vi "Gerador de sinais - Produtor consumidor.vi"() -> ()   [LabVIEW 2019]
doc: "[Covers: REQ08]\n[Covers: REQ04]\n[Covers: REQ05]\n[Covers: REQ06]\n[Covers: REQ03]"
uses:
  Estados - Consumidor.ctl
  Dados consumidor.ctl
  <vilib>/Utility/sysdir.llb/System Directory Type.ctl
  <vilib>/Waveform/WDTOps.llb/WDT Append Waveforms DBL.vi
  <vilib>/Waveform/WDTOps.llb/WDT Waveform Duration DBL.vi
  <vilib>/measure/NI_MABase.lvlib
panel:
  in  "Power":bool
  in  "Concatenar":bool
  in  "Adquirir entre cursores":bool
  in  "Deletar entre cursores":bool
  in  "Concatenar entre cursores":bool
  in  "Fase         º":dbl(slide) caption="Horizontal Slider" min=0.0 max=360.0 step=0.5 scale=0.0..360.0 scale format="%#.6g"
  in  "Offset":dbl(slide) caption="Vertical Slider" min=-10.0 max=10.0 step=0.01 scale=-10.0..10.0 scale format="%#2_2g"
  in  "Forma de onda":T1(ring) caption="Enum"
  in  "Tempo (Segundos)":dbl(knob)=1.0 min=0.0 max=1.0 scale=0.0..1.0
  in  "Abrir arquivo":bool
  in  "Salvar":bool
  out "Edição":waveform(dbl)(graph)
  out "Plot":waveform(dbl)(graph)
  in  "Razão cíclica (%)":dbl(knob)=50.0 min=0.0 max=100.0 step=0.5 scale=0.0..100.0
  in  "Amplitude":dbl(knob)=5.0 min=0.0 max=10.0 step=0.01 scale=0.0..10.0
  in  "Frequência":dbl(knob)=1.0 min=0.0 max=10.0 step=0.01 scale=0.0..10.0
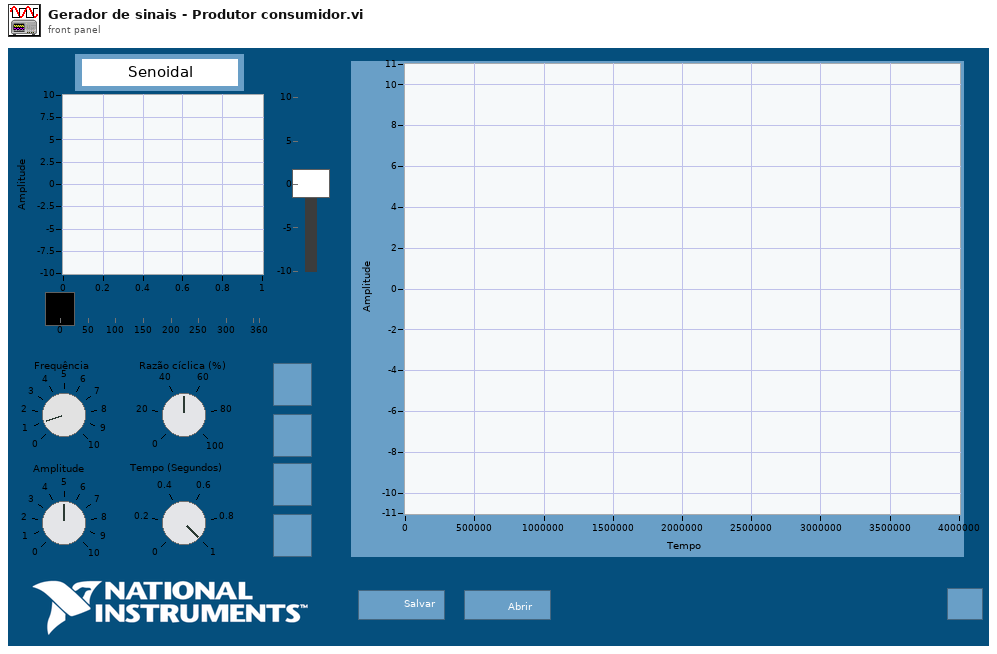
[diagram p1: front panel]
types:
  T1 = enum16{"Senoidal", "Triangular", "Quadrada", "Dente de Serra", "Trapezoidal"}
  T2 = typedef "Estados - Consumidor.ctl" = enum16{"Gerar onda", "Inicialização", "Parada", "Plotar", "Concatenar", "Concatenar - Cursores", "Adquirir entre Cursores", "Deletar entre Cursores", "Salvar onda", "Carregar onda", "Posicionar Cursores"}
  T3 = typedef "Dados consumidor.ctl" = cluster{"Onda gerada":cluster{"onda":waveform(dbl)}, "Onda modificada":cluster{"onda":waveform(dbl)}}
  T4 = typedef "Informações.ctl" = cluster{"Estados":T2, "Amplitude":dbl, "Informação\nde amostragem":cluster{"Fs":dbl, "#s":dbl}, "Frequência":dbl, "Offset":dbl, "Fase (Graus)":dbl, "Razão cíclica (%)":dbl, "Sinal":enum16{"Sine Wave", "Triangle Wave", "Square Wave", "Sawtooth Wave", "Trapezoidal Wave"}}
  T5 = enum8{"Enabled", "Disabled", "Disabled and Grayed Out"}
  T6 = enum16{"Sine Wave", "Triangle Wave", "Square Wave", "Sawtooth Wave", "Trapezoidal Wave"}
  T7 = enum16{"open", "open or create", "create or replace", "create", "open (read-only)"}
  T8 = typedef "System Directory Type.ctl" = i32
  T9 = cluster{"Amostras / s":dbl, "Quantidade\nde amostras":dbl}
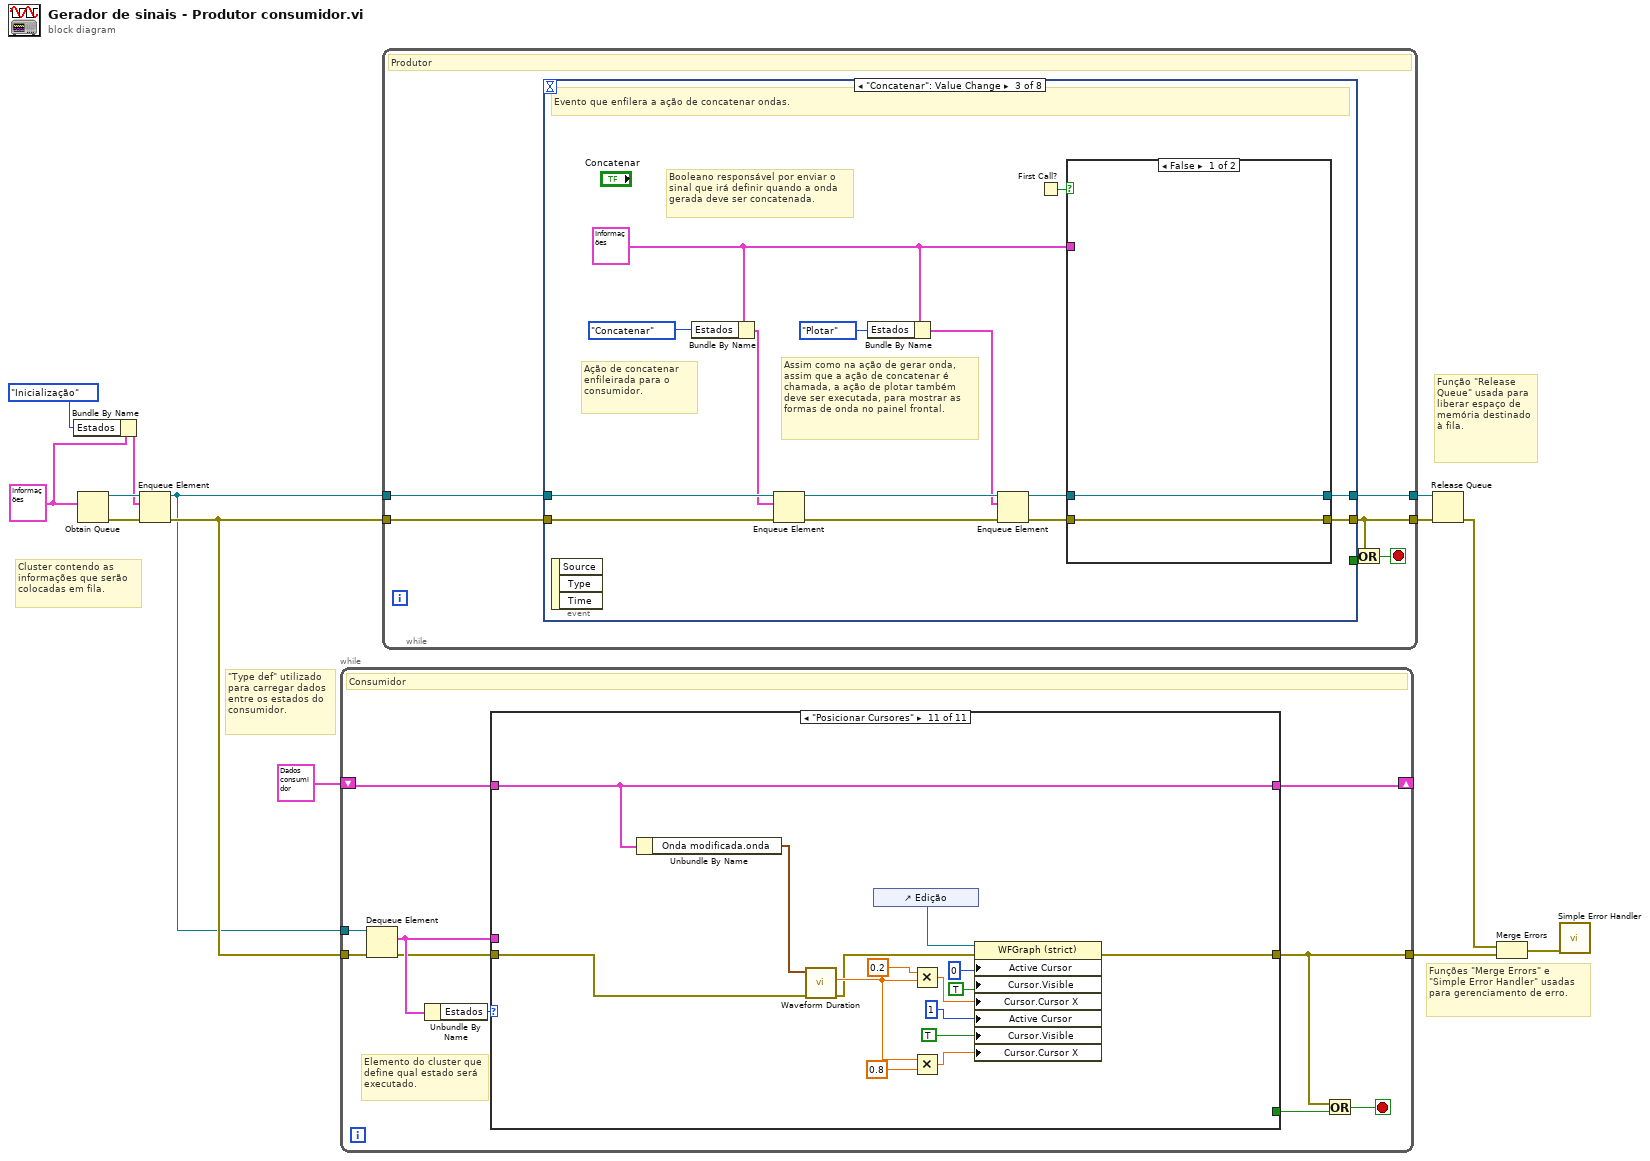
[diagram p0: block diagram]
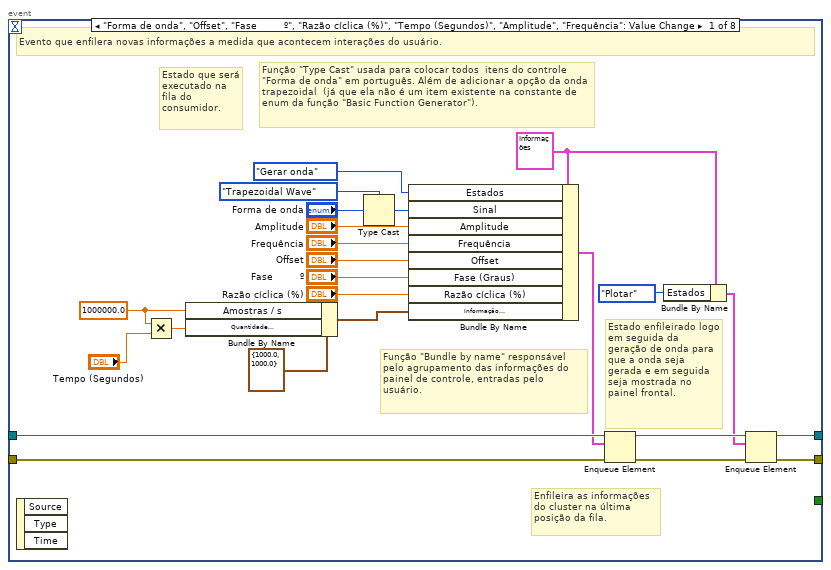
[diagram p2: hidden frame]
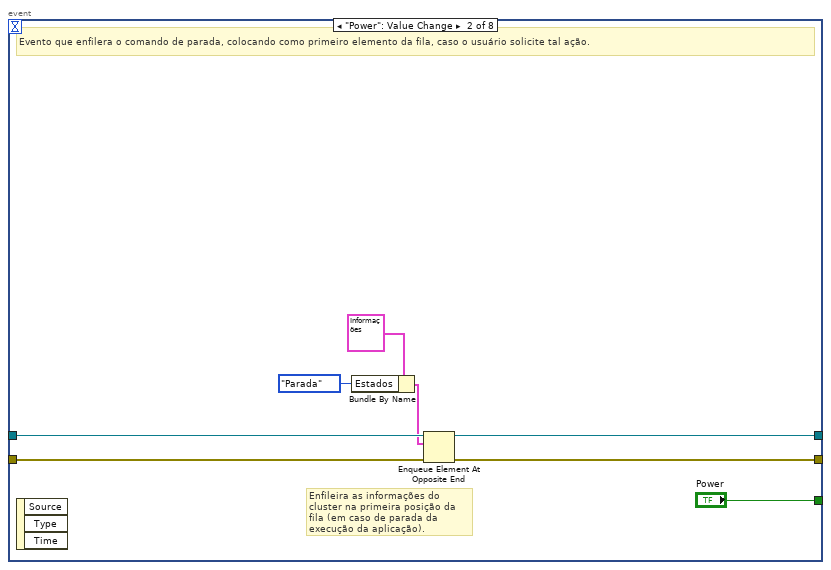
[diagram p3: hidden frame]
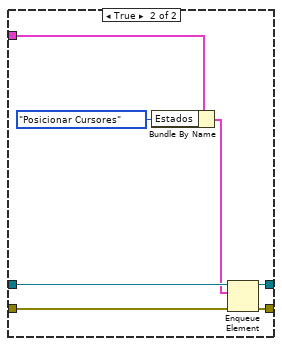
[diagram p4: hidden frame]
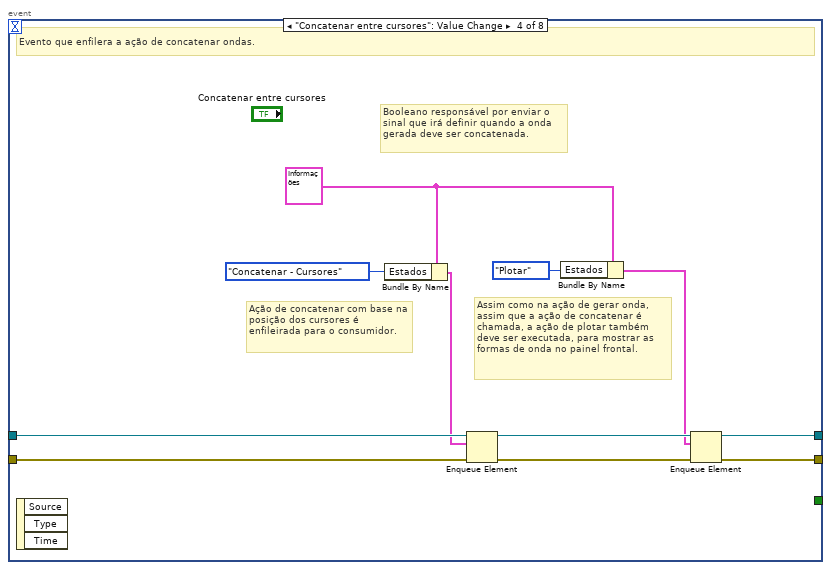
[diagram p5: hidden frame]
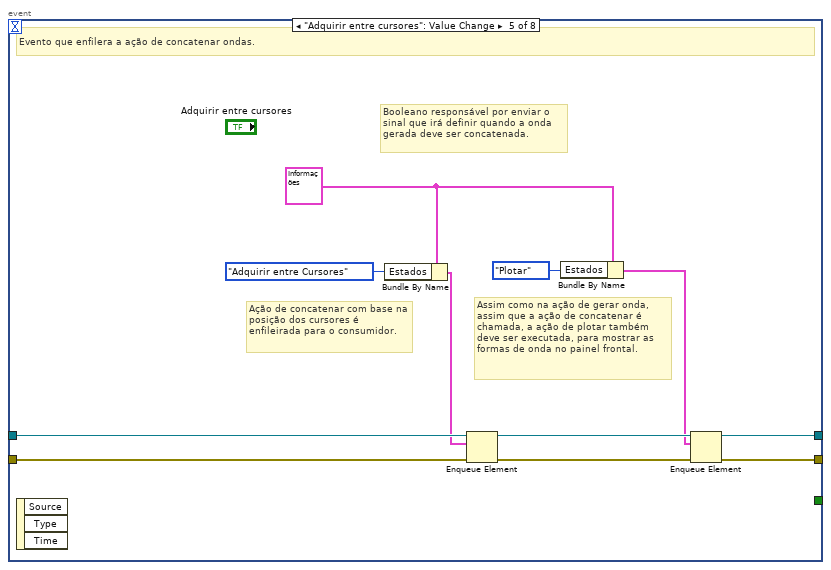
[diagram p6: hidden frame]
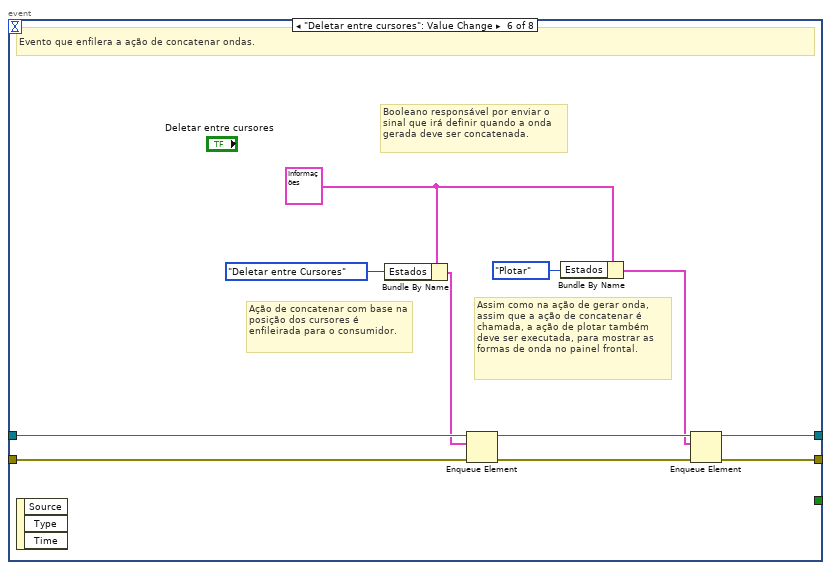
[diagram p7: hidden frame]
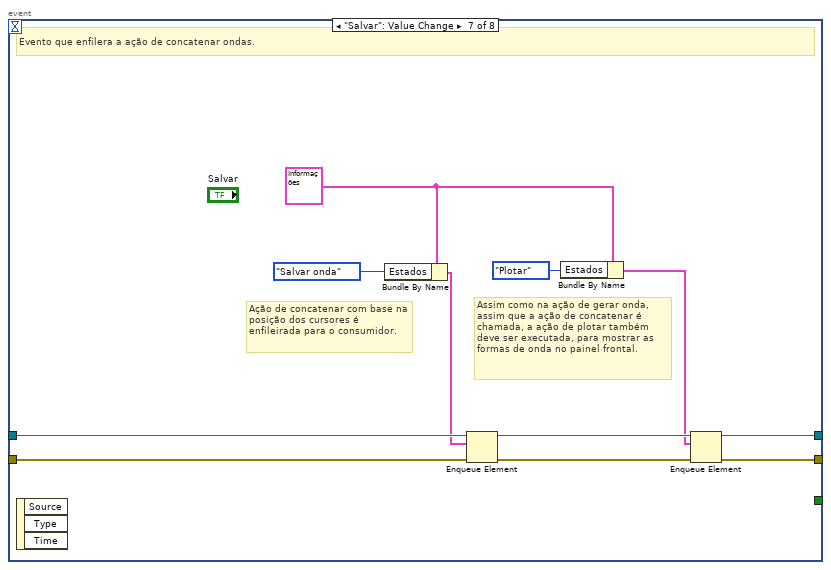
[diagram p8: hidden frame]
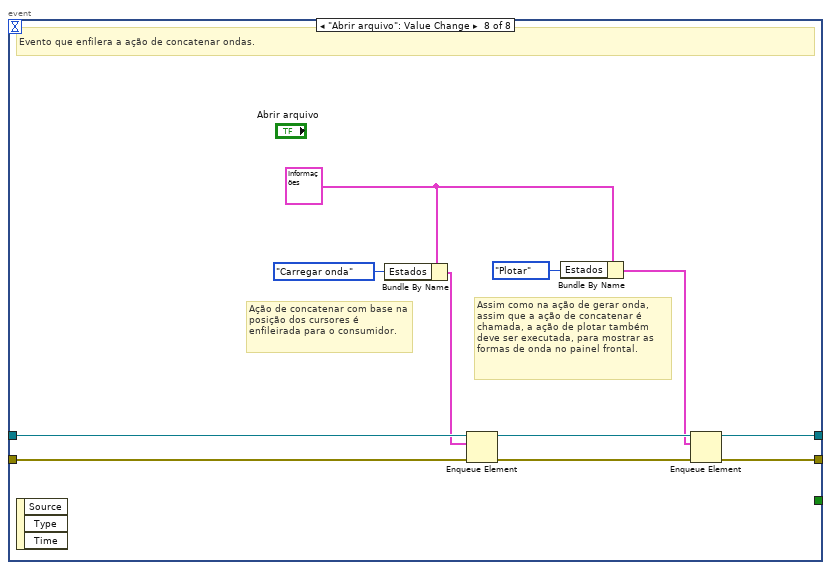
[diagram p9: hidden frame]
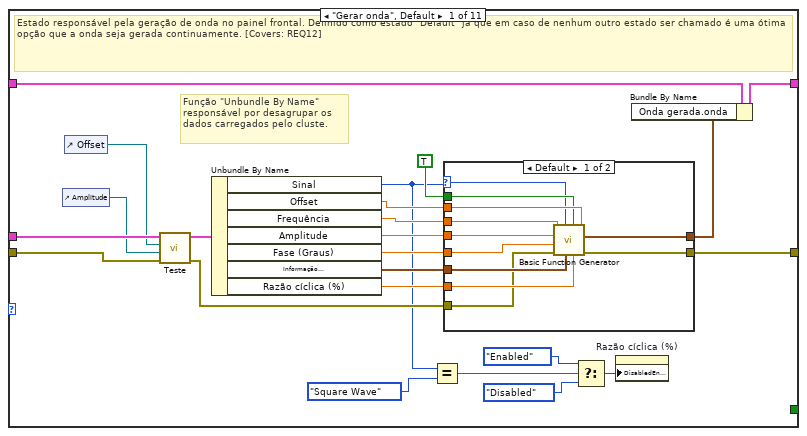
[diagram p10: hidden frame]
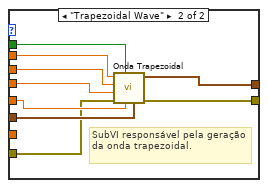
[diagram p11: hidden frame]
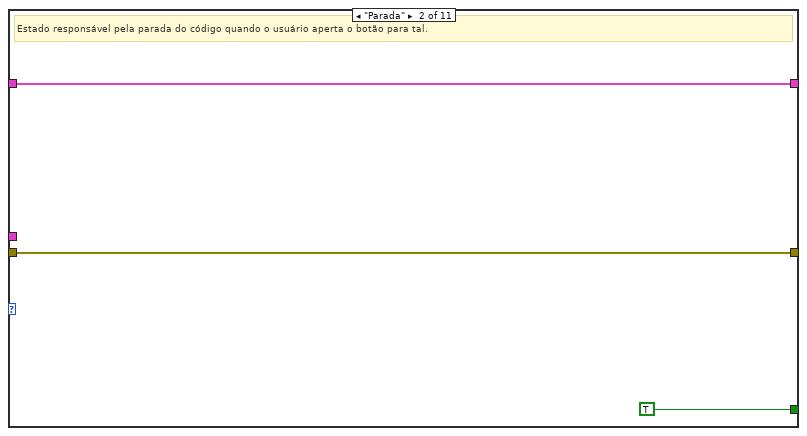
[diagram p12: hidden frame]
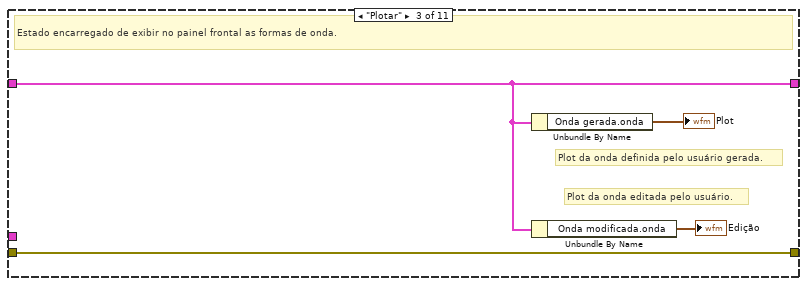
[diagram p13: hidden frame]
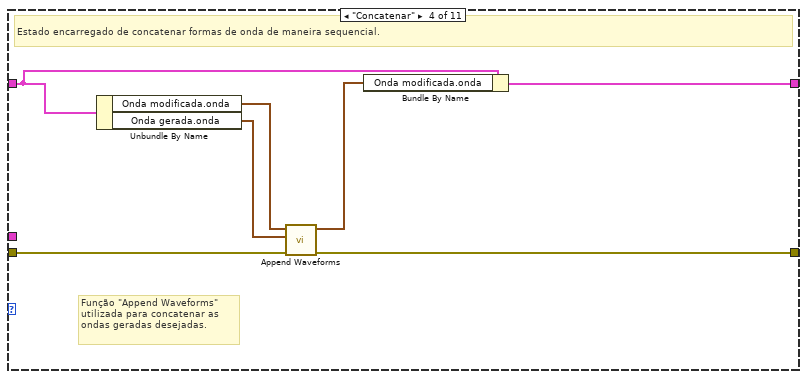
[diagram p14: hidden frame]
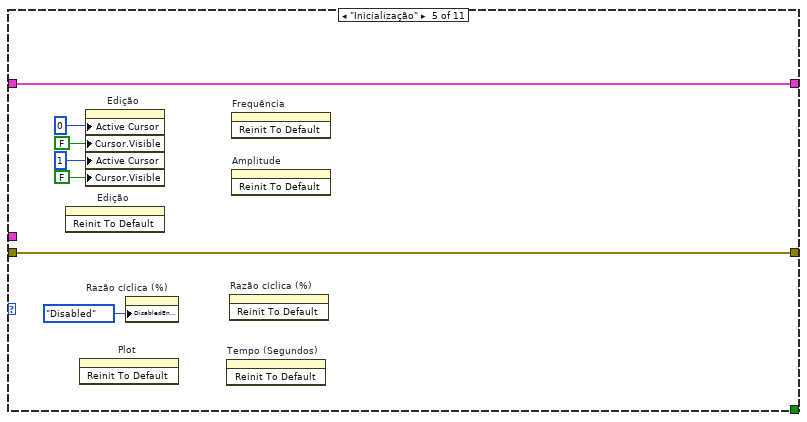
[diagram p15: hidden frame]
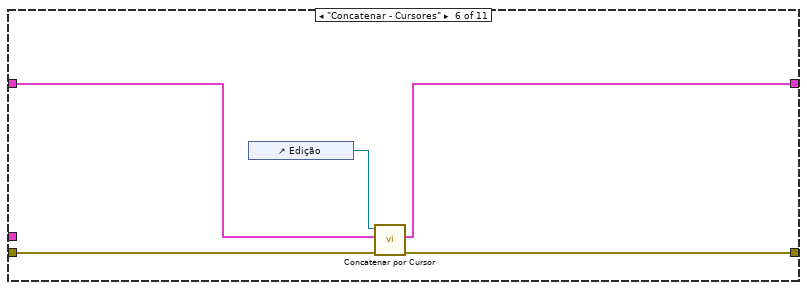
[diagram p16: hidden frame]
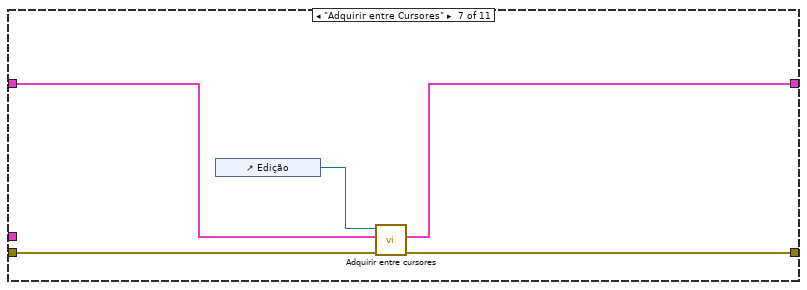
[diagram p17: hidden frame]
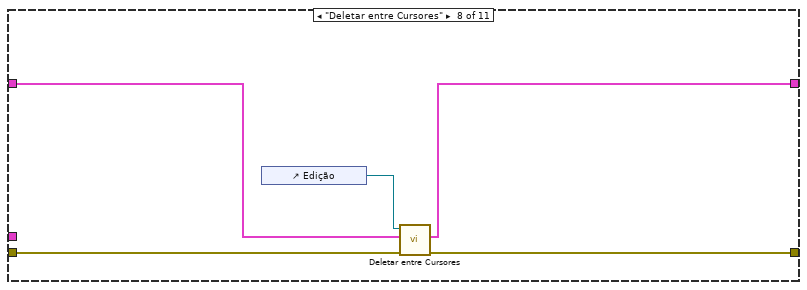
[diagram p18: hidden frame]
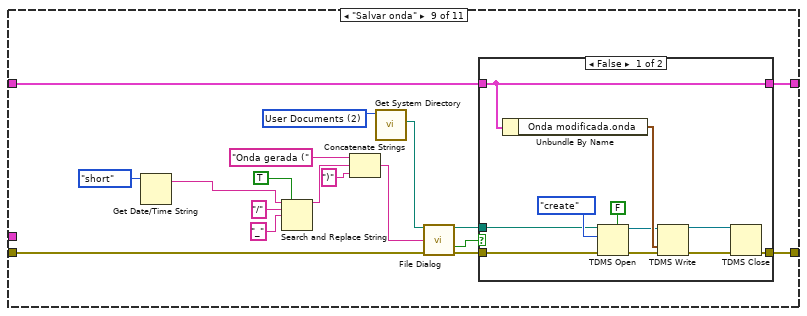
[diagram p19: hidden frame]
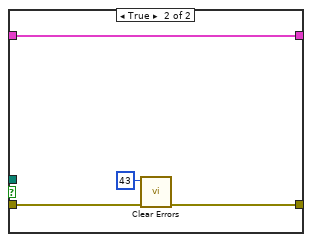
[diagram p20: hidden frame]
diagram:
  w2 = T4 {"Estados"=enum."Gerar onda", "Amplitude"=0.0, "Informação\nde amostragem"={"Fs"=1000.0, "#s"=1000.0}, "Frequência"=0.0, "Offset"=0.0, "Fase (Graus)"=0.0, "Razão cíclica (%)"=0.0, "Sinal"=enum."Sine Wave"}
  # "\"Type def\" utilizado para carregar dados entre os estados do consumidor."
  # "Funções \"Merge Errors\" e \"Simple Error Handler\" usadas para gerenciamento de erro."
  # "Função \"Release Queue\" usada para liberar espaço de memória destinado à fila."
  # "Cluster contendo as informações que serão colocadas em fila."
  n1 = Bundle By Name(cluster=w2, "Estados"=Estados_-_Consumidor."Inicialização") -> (w3:T4)
  n2 = Obtain Queue(element data type=w2) -> (queue out=w5:refnum<queue>, error out=w8:errorcluster)  [unwired: 4 in, 1 out]
  n3 = Enqueue Element(queue=w5, element=w3, error in (no error)=w8) -> (queue out=w4:refnum<queue>, error out=w6:errorcluster)  [unwired: 1 in, 1 out]
  n4 = while {
    tunnel: w4 -> [w16]
    tunnel: [w21] -> w10
    tunnel: w6 -> [w17]
    shift-right: [w15] -> _
    shift-left: T3 {"Onda gerada"={"onda"={"t0"=timestamp(0 s since 1904-01-01), "dt"=1.0, "Y"=[]}}, "Onda modificada"={"onda"={"t0"=timestamp(0 s since 1904-01-01), "dt"=1.0, "Y"=[]}}} ("Cluster 3") -> [w14]
    stop <- w19 stop-if-true
    # "Elemento do cluster que define qual estado será executado."
    # "Consumidor"
    n5 = Dequeue Element(queue=w16, error in (no error)=w17) -> (element=w22:T4, error out=w18:errorcluster)  [unwired: 1 in, 2 out]
    n6 = Unbundle By Name(w22) -> ("Estados"=w23:T2)
    n7 = case shown="\"Posicionar Cursores\"" w23 {
      tunnel: w22 -> [w46 _ _ _ _ _ _ _ _ _ _]
      tunnel: [_ TRUE _ _ _ _ _ _ _ _ _] -> w20
      tunnel: [w38 w67 w70 w74 w86 w90 w96 w98 w106 w137 w165] -> w21
      tunnel: w18 -> [w33 w67 w70 w77 w86 w91 w97 w99 w109 w140 w163]
      tunnel: [w36 w68 w71 w79 w87 w88 w94 w100 w103 w138 w167] -> w15
      tunnel: w14 -> [w37 w68 w71 w80 w87 w89 w95 w101 w107 w139 w167]
      frame "Gerar onda", Default {
        # "Função \"Unbundle By Name\" responsável por desagrupar os dados carregados pelo cluste."
        # "Estado responsável pela geração de onda no painel frontal. Definido como estado \"Default\" já que em caso de nenhum outro estado ser chamado é uma ótima opção que a onda seja gerada continuamente. [Covers: REQ12]"
        n8 = control-ref of="Amplitude"() -> (w31:refnum<vi>)
        n9 = control-ref of="Offset"() -> (w24:refnum<vi>)
        n10 = call "Teste.vi"("error in (no error)"=w33, "Amplitude Refnum"=w31, "Offset Refnum"=w24, 11:w46) -> ("error out"=w32:errorcluster, 3:w34:T4)  [unwired: 6 in]
        n11 = Unbundle By Name(w34) -> ("Sinal"=w25:T6, "Offset"=w45:dbl, "Frequência"=w44:dbl, "Amplitude"=w43:dbl, "Fase (Graus)"=w42:dbl, "Informação\nde amostragem"=w41:cluster{"Fs":dbl, "#s":dbl}, "Razão cíclica (%)"=w40:dbl)
        n12 = Equal?(x=w25, y=T6."Square Wave" ("Sinal")) -> (x = y?=w30:bool)
        n13 = case shown="Default" w25 {
          selector: w25 -> [w49 _]
          tunnel: w45 -> [w57 w60]
          tunnel: w44 -> [w56 w62]
          tunnel: w43 -> [w55 w61]
          tunnel: w42 -> [w54 w65]
          tunnel: w41 -> [w53 w64]
          tunnel: w40 -> [w52 _]
          tunnel: [w51 w63] -> w35
          tunnel: TRUE ("reset signal") -> [w50 w66]
          tunnel: [w48 w58] -> w38
          tunnel: w32 -> [w47 w59]
          frame Default {
            n14 = call <vilib>:"Basic Function Generator.vi"("offset"=w57, "square wave duty cycle (%)"=w52, "reset signal"=w50, "sampling info"=w53, "signal type"=w49, "error in (no error)"=w47, "phase"=w54, "amplitude"=w55, "frequency"=w56) -> ("error out"=w48:errorcluster, "signal out"=w51:waveform(dbl))  [unwired: 1 out]
          }
          frame "Trapezoidal Wave" {
            # "SubVI responsável pela geração da onda trapezoidal."
            n15 = call "Onda Trapezoidal.vi"("Informação\nde amostragem"=w64, "Fase (Graus)"=w65, "Reset do sinal"=w66, "Entrada de erro"=w59, "Amplitude"=w61, "Frequência"=w62, "Offset"=w60) -> ("Saída de erro"=w58:errorcluster, "Saída de sinal"=w63:waveform(dbl))  [unwired: 3 in]
          }
        }
        n16 = Select(t=T5."Enabled" ("Disabled"), s=w30, f=T5."Disabled" ("Disabled")) -> (s? t:f=w29:T5)
        n17 = property on="Razão cíclica (%)" class="Knob (strict)"("DisabledEnum"=w29) -> ()  [unwired: 2 in, 2 out]
        n18 = Bundle By Name(cluster=w37, "Onda gerada.onda"=w35) -> (w36:T3)
      }
      frame "Parada" {
        # "Estado responsável pela parada do código quando o usuário aperta o botão para tal."
      }
      frame "Plotar" {
        # "Plot da onda editada pelo usuário."
        # "Plot da onda definida pelo usuário gerada."
        # "Estado encarregado de exibir no painel frontal as formas de onda."
        n19 = Unbundle By Name(w71) -> ("Onda gerada.onda"=→"Plot":waveform(dbl))
        n20 = Unbundle By Name(w71) -> ("Onda modificada.onda"=→"Edição":waveform(dbl))
      }
      frame "Concatenar" {
        # "Função \"Append Waveforms\" utilizada para concatenar as ondas geradas desejadas."
        # "Estado encarregado de concatenar formas de onda de maneira sequencial."
        n21 = Unbundle By Name(w80) -> ("Onda modificada.onda"=w78:waveform(dbl), "Onda gerada.onda"=w76:waveform(dbl))
        n22 = call-poly <vilib>:"Append Waveforms.vi"("error in (no error)"=w77, "waveform B"=w76, "waveform A"=w78) -> ("error out"=w74:errorcluster, "waveform out"=w75:waveform(dbl))  [unwired: 7 in]
        n23 = Bundle By Name(cluster=w80, "Onda modificada.onda"=w75) -> (w79:T3)
      }
      frame "Inicialização" {
        n24 = invoke on="Edição" class="WFGraph (strict)" method="Reinit To Default"() -> ()  [unwired: 3 in, 3 out]
        n25 = invoke on="Plot" class="WFGraph (strict)" method="Reinit To Default"() -> ()  [unwired: 3 in, 3 out]
        n26 = property on="Edição" class="WFGraph (strict)"("Active Cursor"=u32 0, "Cursor.Visible"=FALSE, "Active Cursor"=u32 1, "Cursor.Visible"=FALSE) -> ()  [unwired: 2 in, 2 out]
        n27 = property on="Razão cíclica (%)" class="Knob (strict)"("DisabledEnum"=T5."Disabled" ("Disabled")) -> ()  [unwired: 2 in, 2 out]
        n28 = invoke on="Tempo (Segundos)" class="Knob (strict)" method="Reinit To Default"() -> ()  [unwired: 3 in, 3 out]
        n29 = invoke on="Razão cíclica (%)" class="Knob (strict)" method="Reinit To Default"() -> ()  [unwired: 3 in, 3 out]
        n30 = invoke on="Frequência" class="Knob (strict)" method="Reinit To Default"() -> ()  [unwired: 3 in, 3 out]
        n31 = invoke on="Amplitude" class="Knob (strict)" method="Reinit To Default"() -> ()  [unwired: 3 in, 3 out]
      }
      frame "Concatenar - Cursores" {
        n32 = control-ref of="Edição"() -> (w92:refnum<vi>)
        n33 = call "Concatenar por Cursor.vi"("error in"=w91, "Cluster 3"=w89, "WaveformGraph in"=w92) -> ("error out"=w90:errorcluster, "output cluster"=w88:T3)  [unwired: 7 in]
      }
      frame "Adquirir entre Cursores" {
        n34 = control-ref of="Edição"() -> (w93:refnum<vi>)
        n35 = call "Adquirir entre cursores.vi"("error in"=w97, "Input Cluster"=w95, "WaveformGraph in"=w93) -> ("error out"=w96:errorcluster, "Output Cluster"=w94:T3)  [unwired: 7 in]
      }
      frame "Deletar entre Cursores" {
        n36 = control-ref of="Edição"() -> (w102:refnum<vi>)
        n37 = call "Deletar entre Cursores.vi"("error in"=w99, "Cluster 3"=w101, "WaveformGraph in"=w102) -> ("error out"=w98:errorcluster, "output cluster"=w100:T3)  [unwired: 7 in]
      }
      frame "Salvar onda" {
        w110 = T8 2 items=["User Home"=0, "User Desktop"=1, "User Documents"=2, "User Application Data"=3, "User Preferences"=4, "User Temporary"=5, "Public Documents"=6, "Public Application Data"=7, "Public Preferences"=8, "Public Cache"=13, "System Core Libraries"=9, "System Installed Libraries"=10, "Application Files"=11, "Boot Volume Root"=12] ("system directory type")
        n38 = Get Date/Time String(date format (0)=enum16{"short", "long", "abbreviated"}."short") -> (date string=w115:string)  [unwired: 2 in, 1 out]
        n39 = Search and Replace String(replace all?=TRUE ("replace all? (F)"), input string=w115, search string="/", replace string="_" ("replace string (\"\")")) -> (result string=w120:string)  [unwired: 4 in, 3 out]
        n40 = Concatenate Strings("Onda gerada (" ("string"), w120, ")" ("string")) -> (w112:string)
        n41 = call <vilib>:"Get System Directory.vi"("system directory type"=w110) -> ("system directory"=w111:path)  [unwired: 10 in]
        n42 = call "File Dialog"("start path"=w111, "default name"=w112, "error in"=w109) -> ("selected path"=w108:path, "cancelled"=w105:bool, "error out"=w104:errorcluster)  [unwired: 9 in, 1 out]
        n43 = case shown="False" w105 {
          tunnel: w108 -> [w129 _]
          tunnel: w107 -> [w121 w135]
          tunnel: [w124 w132] -> w106
          tunnel: w104 -> [w122 w133]
          tunnel: [w121 w135] -> w103
          frame False {
            n44 = Unbundle By Name(w121) -> ("Onda modificada.onda"=w128:waveform(dbl))
            n45 = TDMS Open(5:FALSE ("create index file? (T)"), 8:w122, 10:T7."create" ("operation (0:open)"), 11:w129) -> (0:w127:errorcluster, 3:w126:refnum<k34>)  [unwired: 3 in]
            n46 = TDMS Write(0:w126, 9:w128, 11:w127) -> (4:w123:refnum<k34>, 15:w125:errorcluster)  [unwired: 3 in, 2 out]
            n47 = TDMS Close(8:w125, 11:w123) -> (0:w124:errorcluster)  [unwired: 1 out]
          }
          frame True {
            n48 = call <vilib>:"Clear Errors.vi"("error in (no error)"=w133, "specific error code to clear (0: all)"=43) -> ("error out"=w132:errorcluster)  [unwired: 4 in, 1 out]
          }
        }
      }
      frame "Carregar onda" {
        w143 = T8 2 items=["User Home"=0, "User Desktop"=1, "User Documents"=2, "User Application Data"=3, "User Preferences"=4, "User Temporary"=5, "Public Documents"=6, "Public Application Data"=7, "Public Preferences"=8, "Public Cache"=13, "System Core Libraries"=9, "System Installed Libraries"=10, "Application Files"=11, "Boot Volume Root"=12] ("system directory type")
        n49 = call <vilib>:"Get System Directory.vi"("system directory type"=w143) -> ("system directory"=w144:path)  [unwired: 10 in]
        n50 = call "File Dialog2"("start path"=w144, "error in"=w140) -> ("selected path"=w141:path, "cancelled"=w136:bool, "error out"=w142:errorcluster)  [unwired: 10 in, 1 out]
        n51 = case shown="False" w136 {
          tunnel: w142 -> [w145 w160]
          tunnel: w141 -> [w155 _]
          tunnel: w139 -> [w150 w158]
          tunnel: [w149 w158] -> w138
          tunnel: [w146 w159] -> w137
          frame False {
            n52 = TDMS Open(5:FALSE ("create index file? (T)"), 8:w145, 10:T7."open (read-only)" ("operation (0:open)"), 11:w155) -> (0:w154:errorcluster, 3:w153:refnum<k34>)  [unwired: 3 in]
            n53 = TDMS Read(0:w153, 11:w154, 12:waveform(dbl) {"t0"=timestamp(0 s since 1904-01-01), "dt"=1.0, "Y"=[]} ("Onda modificada.onda")) -> (4:w151:refnum<k34>, 10:w147:waveform(dbl), 15:w152:errorcluster)  [unwired: 5 in, 3 out]
            n54 = Bundle By Name(cluster=w150, "Onda modificada.onda"=w147) -> (w149:T3)
            n55 = TDMS Close(8:w152, 11:w151) -> (0:w146:errorcluster)  [unwired: 1 out]
          }
          frame True {
            n56 = call <vilib>:"Clear Errors.vi"("error in (no error)"=w160, "specific error code to clear (0: all)"=43) -> ("error out"=w159:errorcluster)  [unwired: 4 in, 1 out]
          }
        }
      }
      frame "Posicionar Cursores" {
        n57 = Unbundle By Name(w167) -> ("Onda modificada.onda"=w166:waveform(dbl))
        n58 = call-poly <vilib>:"Waveform Duration.vi"("error in (no error)"=w163, "waveform in"=w166) -> ("error out"=w164:errorcluster, "duration"=w174:dbl)  [unwired: 7 in, 1 out]
        n59 = control-ref of="Edição"() -> (w162:refnum<vi>)
        n60 = Multiply(x=0.2 ("y"), y=w174) -> (x*y=w176:dbl)
        n61 = Multiply(x=w174, y=0.8) -> (x*y=w175:dbl)
        n62 = property on="Property Node" class="WFGraph (strict)"(reference=w162, error in=w164, "Active Cursor"=u32 0, "Cursor.Visible"=TRUE, "Cursor.Cursor X"=w176, "Active Cursor"=u32 1, "Cursor.Visible"=TRUE, "Cursor.Cursor X"=w175) -> (error out=w165:errorcluster)  [unwired: 1 out]
      }
    }
    n63 = Or(x=w21, y=w20) -> (x .or. y?=w19:bool)
  }
  n64 = while {
    tunnel: w4 -> [w182]
    tunnel: [w178] -> w13
    tunnel: w6 -> [w181]
    tunnel: [w177] -> w12
    stop <- w179 stop-if-true
    # "Produtor"
    n65 = event shown="[2] \"Concatenar\": Value Change" {
      selector: _ -> [_ _ _ _ _ _ _ _]
      dyn-events: _ -> [_ _ _ _ _ _ _ _]
      timeout: _ -> [_ _ _ _ _ _ _ _]
      tunnel: w182 -> [w206 w212 w226 w245 w256 w267 w278 w289]
      tunnel: w181 -> [w205 w214 w228 w248 w259 w270 w281 w292]
      tunnel: [w197 w213 w216 w246 w257 w268 w279 w290] -> w177
      tunnel: [_ "Power" _ _ _ _ _ _] -> w180
      tunnel: [w195 w210 w215 w243 w254 w265 w276 w287] -> w178
      event "Forma de onda", "Offset", "Fase         º", "Razão cíclica (%)", "Tempo (Segundos)", "Amplitude", "Frequência": Value Change {
        w187 = 1000000.0 ("Quantidade\nde amostras")
        w194 = T4 {"Estados"=enum."Gerar onda", "Amplitude"=0.0, "Informação\nde amostragem"={"Fs"=1000.0, "#s"=1000.0}, "Frequência"=0.0, "Offset"=0.0, "Fase (Graus)"=0.0, "Razão cíclica (%)"=0.0, "Sinal"=enum."Sine Wave"}
        # "Estado enfileirado logo em seguida da geração de onda para que a onda seja gerada e em seguida seja mostrada no painel frontal."
        # "Função \"Type Cast\" usada para colocar todos  itens do controle \"Forma de onda\" em português. Além de adicionar a opção da onda trapezoidal  (já que ela não é um item existente na constante de enum da função \"Basic Function Generator\")."
        # "Estado que será executado na fila do consumidor."
        # "Enfileira as informações do cluster na última posição da fila."
        # "Função \"Bundle by name\" responsável pelo agrupamento das informações do painel de controle, entradas pelo usuário."
        # "Evento que enfilera novas informações a medida que acontecem interações do usuário."
        n66 = event-data() -> ()  [unwired: 1 in, 3 out]
        n67 = Multiply(x=w187, y="Tempo (Segundos)") -> (x*y=w188:dbl)
        n68 = Bundle By Name(cluster=T9 {"Amostras / s"=1000.0, "Quantidade\nde amostras"=1000.0} ("Informação\nde amostragem"), "Amostras / s"=w187, "Quantidade\nde amostras"=w188) -> (w189:T9)
        n69 = Type Cast(type=T6."Trapezoidal Wave" ("Forma de onda"), x="Forma de onda") -> (*(type *) &x=w198:T6)
        n70 = Bundle By Name(cluster=w194, "Estados"=Estados_-_Consumidor."Gerar onda", "Sinal"=w198, "Amplitude"="Amplitude", "Frequência"="Frequência", "Offset"="Offset", "Fase (Graus)"="Fase         º", "Razão cíclica (%)"="Razão cíclica (%)", "Informação\nde amostragem"=w189) -> (w200:T4)
        n71 = Enqueue Element(queue=w206, element=w200, error in (no error)=w205) -> (queue out=w196:refnum<queue>, error out=w204:errorcluster)  [unwired: 1 in, 1 out]
        n72 = Bundle By Name(cluster=w194, "Estados"=Estados_-_Consumidor."Plotar") -> (w193:T4)
        n73 = Enqueue Element(queue=w196, element=w193, error in (no error)=w204) -> (queue out=w195:refnum<queue>, error out=w197:errorcluster)  [unwired: 1 in, 1 out]
      }
      event "Power": Value Change {
        # "Enfileira as informações do cluster na primeira posição da fila (em caso de parada da execução da aplicação)."
        # "Evento que enfilera o comando de parada, colocando como primeiro elemento da fila, caso o usuário solicite tal ação."
        n74 = event-data() -> ()  [unwired: 1 in, 3 out]
        n75 = Bundle By Name(cluster=T4 {"Estados"=enum."Gerar onda", "Amplitude"=0.0, "Informação\nde amostragem"={"Fs"=1000.0, "#s"=1000.0}, "Frequência"=0.0, "Offset"=0.0, "Fase (Graus)"=0.0, "Razão cíclica (%)"=0.0, "Sinal"=enum."Sine Wave"}, "Estados"=Estados_-_Consumidor."Parada") -> (w211:T4)
        n76 = Enqueue Element At Opposite End(queue=w212, element=w211, error in (no error)=w214) -> (queue out=w210:refnum<queue>, error out=w213:errorcluster)  [unwired: 1 in, 1 out]
      }
      event "Concatenar": Value Change {
        w219 = T4 {"Estados"=enum."Gerar onda", "Amplitude"=0.0, "Informação\nde amostragem"={"Fs"=1000.0, "#s"=1000.0}, "Frequência"=0.0, "Offset"=0.0, "Fase (Graus)"=0.0, "Razão cíclica (%)"=0.0, "Sinal"=enum."Sine Wave"}
        # "Assim como na ação de gerar onda, assim que a ação de concatenar é chamada, a ação de plotar também deve ser executada, para mostrar as formas de onda no painel frontal."
        # "Ação de concatenar enfileirada para o consumidor."
        # "Booleano responsável por enviar o sinal que irá definir quando a onda gerada deve ser concatenada."
        # "Evento que enfilera a ação de concatenar ondas."
        n77 = event-data() -> ()  [unwired: 1 in, 3 out]
        n78 = Bundle By Name(cluster=w219, "Estados"=Estados_-_Consumidor."Concatenar") -> (w224:T4)
        n79 = Enqueue Element(queue=w226, element=w224, error in (no error)=w228) -> (queue out=w225:refnum<queue>, error out=w227:errorcluster)  [unwired: 1 in, 1 out]
        n80 = Bundle By Name(cluster=w219, "Estados"=Estados_-_Consumidor."Plotar") -> (w223:T4)
        n81 = Enqueue Element(queue=w225, element=w223, error in (no error)=w227) -> (queue out=w218:refnum<queue>, error out=w217:errorcluster)  [unwired: 1 in, 1 out]
        n82 = First Call?() -> (First Call?: T/F=w220:bool)
        n83 = case shown="False" w220 {
          tunnel: w219 -> [_ w236]
          tunnel: w218 -> [w230 w235]
          tunnel: w217 -> [w229 w234]
          tunnel: [w229 w233] -> w216
          tunnel: [w230 w232] -> w215
          frame False {
          }
          frame True {
            n84 = Bundle By Name(cluster=w236, "Estados"=Estados_-_Consumidor."Posicionar Cursores") -> (w231:T4)
            n85 = Enqueue Element(queue=w235, element=w231, error in (no error)=w234) -> (queue out=w232:refnum<queue>, error out=w233:errorcluster)  [unwired: 1 in, 1 out]
          }
        }
      }
      event "Concatenar entre cursores": Value Change {
        w240 = T4 {"Estados"=enum."Gerar onda", "Amplitude"=0.0, "Informação\nde amostragem"={"Fs"=1000.0, "#s"=1000.0}, "Frequência"=0.0, "Offset"=0.0, "Fase (Graus)"=0.0, "Razão cíclica (%)"=0.0, "Sinal"=enum."Sine Wave"}
        # "Assim como na ação de gerar onda, assim que a ação de concatenar é chamada, a ação de plotar também deve ser executada, para mostrar as formas de onda no painel frontal."
        # "Ação de concatenar com base na posição dos cursores é enfileirada para o consumidor."
        # "Booleano responsável por enviar o sinal que irá definir quando a onda gerada deve ser concatenada."
        # "Evento que enfilera a ação de concatenar ondas."
        n86 = event-data() -> ()  [unwired: 1 in, 3 out]
        n87 = Bundle By Name(cluster=w240, "Estados"=Estados_-_Consumidor."Concatenar - Cursores") -> (w242:T4)
        n88 = Enqueue Element(queue=w245, element=w242, error in (no error)=w248) -> (queue out=w244:refnum<queue>, error out=w247:errorcluster)  [unwired: 1 in, 1 out]
        n89 = Bundle By Name(cluster=w240, "Estados"=Estados_-_Consumidor."Plotar") -> (w241:T4)
        n90 = Enqueue Element(queue=w244, element=w241, error in (no error)=w247) -> (queue out=w243:refnum<queue>, error out=w246:errorcluster)  [unwired: 1 in, 1 out]
      }
      event "Adquirir entre cursores": Value Change {
        w251 = T4 {"Estados"=enum."Gerar onda", "Amplitude"=0.0, "Informação\nde amostragem"={"Fs"=1000.0, "#s"=1000.0}, "Frequência"=0.0, "Offset"=0.0, "Fase (Graus)"=0.0, "Razão cíclica (%)"=0.0, "Sinal"=enum."Sine Wave"}
        # "Assim como na ação de gerar onda, assim que a ação de concatenar é chamada, a ação de plotar também deve ser executada, para mostrar as formas de onda no painel frontal."
        # "Ação de concatenar com base na posição dos cursores é enfileirada para o consumidor."
        # "Booleano responsável por enviar o sinal que irá definir quando a onda gerada deve ser concatenada."
        # "Evento que enfilera a ação de concatenar ondas."
        n91 = event-data() -> ()  [unwired: 1 in, 3 out]
        n92 = Bundle By Name(cluster=w251, "Estados"=Estados_-_Consumidor."Adquirir entre Cursores") -> (w253:T4)
        n93 = Enqueue Element(queue=w256, element=w253, error in (no error)=w259) -> (queue out=w255:refnum<queue>, error out=w258:errorcluster)  [unwired: 1 in, 1 out]
        n94 = Bundle By Name(cluster=w251, "Estados"=Estados_-_Consumidor."Plotar") -> (w252:T4)
        n95 = Enqueue Element(queue=w255, element=w252, error in (no error)=w258) -> (queue out=w254:refnum<queue>, error out=w257:errorcluster)  [unwired: 1 in, 1 out]
      }
      event "Deletar entre cursores": Value Change {
        w262 = T4 {"Estados"=enum."Gerar onda", "Amplitude"=0.0, "Informação\nde amostragem"={"Fs"=1000.0, "#s"=1000.0}, "Frequência"=0.0, "Offset"=0.0, "Fase (Graus)"=0.0, "Razão cíclica (%)"=0.0, "Sinal"=enum."Sine Wave"}
        # "Assim como na ação de gerar onda, assim que a ação de concatenar é chamada, a ação de plotar também deve ser executada, para mostrar as formas de onda no painel frontal."
        # "Ação de concatenar com base na posição dos cursores é enfileirada para o consumidor."
        # "Booleano responsável por enviar o sinal que irá definir quando a onda gerada deve ser concatenada."
        # "Evento que enfilera a ação de concatenar ondas."
        n96 = event-data() -> ()  [unwired: 1 in, 3 out]
        n97 = Bundle By Name(cluster=w262, "Estados"=Estados_-_Consumidor."Deletar entre Cursores") -> (w264:T4)
        n98 = Enqueue Element(queue=w267, element=w264, error in (no error)=w270) -> (queue out=w266:refnum<queue>, error out=w269:errorcluster)  [unwired: 1 in, 1 out]
        n99 = Bundle By Name(cluster=w262, "Estados"=Estados_-_Consumidor."Plotar") -> (w263:T4)
        n100 = Enqueue Element(queue=w266, element=w263, error in (no error)=w269) -> (queue out=w265:refnum<queue>, error out=w268:errorcluster)  [unwired: 1 in, 1 out]
      }
      event "Salvar": Value Change {
        w273 = T4 {"Estados"=enum."Gerar onda", "Amplitude"=0.0, "Informação\nde amostragem"={"Fs"=1000.0, "#s"=1000.0}, "Frequência"=0.0, "Offset"=0.0, "Fase (Graus)"=0.0, "Razão cíclica (%)"=0.0, "Sinal"=enum."Sine Wave"}
        # "Assim como na ação de gerar onda, assim que a ação de concatenar é chamada, a ação de plotar também deve ser executada, para mostrar as formas de onda no painel frontal."
        # "Ação de concatenar com base na posição dos cursores é enfileirada para o consumidor."
        # "Evento que enfilera a ação de concatenar ondas."
        n101 = event-data() -> ()  [unwired: 1 in, 3 out]
        n102 = Bundle By Name(cluster=w273, "Estados"=Estados_-_Consumidor."Salvar onda") -> (w275:T4)
        n103 = Enqueue Element(queue=w278, element=w275, error in (no error)=w281) -> (queue out=w277:refnum<queue>, error out=w280:errorcluster)  [unwired: 1 in, 1 out]
        n104 = Bundle By Name(cluster=w273, "Estados"=Estados_-_Consumidor."Plotar") -> (w274:T4)
        n105 = Enqueue Element(queue=w277, element=w274, error in (no error)=w280) -> (queue out=w276:refnum<queue>, error out=w279:errorcluster)  [unwired: 1 in, 1 out]
      }
      event "Abrir arquivo": Value Change {
        w284 = T4 {"Estados"=enum."Gerar onda", "Amplitude"=0.0, "Informação\nde amostragem"={"Fs"=1000.0, "#s"=1000.0}, "Frequência"=0.0, "Offset"=0.0, "Fase (Graus)"=0.0, "Razão cíclica (%)"=0.0, "Sinal"=enum."Sine Wave"}
        # "Assim como na ação de gerar onda, assim que a ação de concatenar é chamada, a ação de plotar também deve ser executada, para mostrar as formas de onda no painel frontal."
        # "Ação de concatenar com base na posição dos cursores é enfileirada para o consumidor."
        # "Evento que enfilera a ação de concatenar ondas."
        n106 = event-data() -> ()  [unwired: 1 in, 3 out]
        n107 = Bundle By Name(cluster=w284, "Estados"=Estados_-_Consumidor."Carregar onda") -> (w286:T4)
        n108 = Enqueue Element(queue=w289, element=w286, error in (no error)=w292) -> (queue out=w288:refnum<queue>, error out=w291:errorcluster)  [unwired: 1 in, 1 out]
        n109 = Bundle By Name(cluster=w284, "Estados"=Estados_-_Consumidor."Plotar") -> (w285:T4)
        n110 = Enqueue Element(queue=w288, element=w285, error in (no error)=w291) -> (queue out=w287:refnum<queue>, error out=w290:errorcluster)  [unwired: 1 in, 1 out]
      }
    }
    n111 = Or(x=w177, y=w180) -> (x .or. y?=w179:bool)
  }
  n112 = Release Queue(queue=w13, error in (no error)=w12) -> (error out=w11:errorcluster)  [unwired: 1 in, 2 out]
  n113 = Merge Errors(w11, w10) -> (w9:errorcluster)
  n114 = call <vilib>:"Simple Error Handler.vi"("error in (no error)"=w9) -> ()  [unwired: 4 in, 5 out]
